vi "Send Headers.vi"(8 "error in (no error)":errorcluster, 9 "Stream in":refnum<k5>, 10 "Content-Length":i64, 11 "Streamable Response in":refnum<class "Streamable Response.lvclass">) -> (0 "error out":errorcluster, 1 "Stream out":refnum<k5>, 3 "Streamable Response out":refnum<class "Streamable Response.lvclass">)   [LabVIEW 2020, in "HTTP Utils.lvlib" / "Streamable Response.lvclass"]
uses:
  Streamable Response.lvclass
  C:/dev/lv20CE/relink/lv-http-util/HTTP Utils/Response/Response.lvclass
  lv-stream/stream/Stream/Stream.lvclass/Stream.ctl
  lv-stream/stream/Stream/Dispatch Sniffer Data.vi
  lv-stream/stream/Stream/Prepared.vi
  lv-stream/stream/Endpoint/Cast Sniffer Callback.vi
  lv-stream/stream/Error Bad State.vi
  <vilib>/Utility/error.llb/Error Cluster From Error Code.vi
  lv-stream/stream/Stream/Stream.lvclass
  Streamable Response.lvclass/Streamable Response.ctl
  Response/Response.lvclass
  HTTP Utils.lvlib
  C:/dev/lv20CE/relink/lv-http-util/HTTP Utils/Streamable Response/Streamable Response.lvclass
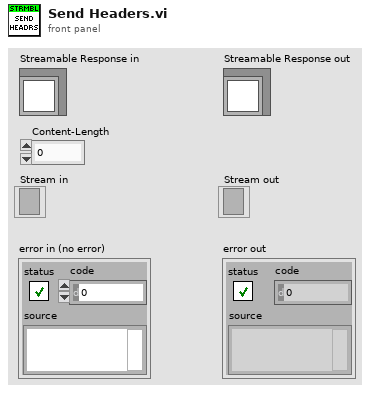
[diagram p1: front panel]
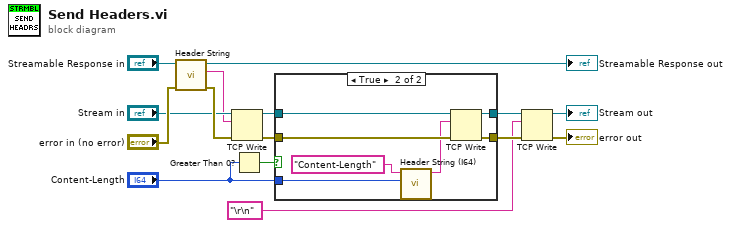
[diagram p0: block diagram]
diagram:
  n1 = call "Header String.vi"("error in (no error)"="error in (no error)", "Response in"="Streamable Response in") -> ("error out"=w15:errorcluster, "Header String"=w6:string, "Response out"=→"Streamable Response out":refnum<class "Streamable Response.lvclass">)  [unwired: 7 in]
  n2 = TCP Write(connection ID="Stream in", data in=w6, error in (no error)=w15) -> (connection ID out=w8:refnum<k5>, error out=w7:errorcluster)  [unwired: 1 in, 1 out]
  n3 = Greater Than 0?(x="Content-Length") -> (x > 0?=w11:bool)
  n4 = case shown="True" w11 {
    tunnel: "Content-Length" -> [_ w24]
    tunnel: w7 -> [w16 w22]
    tunnel: w8 -> [w17 w20]
    tunnel: [w17 w19] -> w3
    tunnel: [w16 w18] -> w5
    frame False {
    }
    frame True {
      n5 = call "Header String (I64).vi"("Value"=w24, "Name"="Content-Length") -> ("Header"=w21:string)  [unwired: 9 in]
      n6 = TCP Write(connection ID=w20, data in=w21, error in (no error)=w22) -> (connection ID out=w19:refnum<k5>, error out=w18:errorcluster)  [unwired: 1 in, 1 out]
    }
  }
  n7 = TCP Write(connection ID=w3, data in="\r\n" ("string"), error in (no error)=w5) -> (connection ID out=→"Stream out":refnum<k5>, error out=→"error out":errorcluster)  [unwired: 1 in, 1 out]
